vi "ini_read_string.vi"(7 "section":string, 8 "error in":errorcluster, 9 "default value":string, 10 "key":string, 11 "refnum in":T1) -> (0 "error out":errorcluster, 1 "value":string, 2 "found?":bool, 3 "refnum out":T1)   [LabVIEW 2020]
uses:
  <vilib>/Utility/config.llb/Config Data RefNum.ctl
  <vilib>/Utility/config.llb/Read Key (String).vi
  <vilib>/Utility/config.llb/NI_LVConfig.lvlib
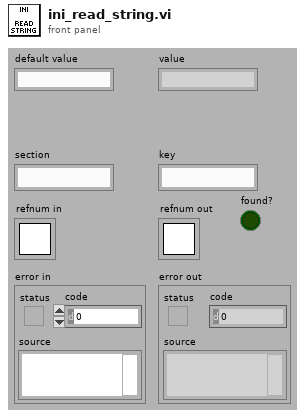
[diagram p1: front panel]
types:
  T1 = typedef "NI_LVConfig.lvlib/Config Data RefNum.ctl" = refnum<k1>
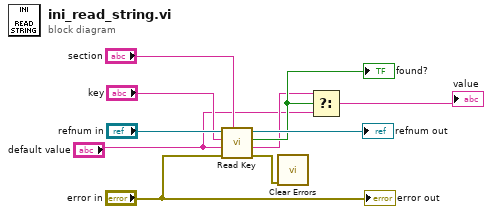
[diagram p0: block diagram]
diagram:
  n1 = call-poly <vilib>:"Read Key.vi"("section"="section", "error in (no error)"="error in", "default value"="default value", "key"="key", "refnum"="refnum in") -> ("error out"=w5:errorcluster, "value"=w3:string, "found?"=w4:bool, "refnum out"=→"refnum out":T1)  [unwired: 3 in]
  "found?" <- w4
  n2 = call <vilib>:"Clear Errors.vi"("error in (no error)"=w5) -> ()  [unwired: 5 in, 2 out]
  n3 = Select(t=w3, s=w4, f="default value") -> (s? t:f=→"value":string)
  "error out" <- "error in"
